vi "Modified Bartlett-Hanning Window.vi"   [LabVIEW 2020, in "NI_AALPro.lvlib"]
doc: "Applies a modified Bartlett-Hanning window to the input signal <B>X</B>. Wire data to the <B>X</B> input to determine the polymorphic instance to use or manually select the instance."
uses:
  <vilib>/Analysis/NI_AALPro.lvlib
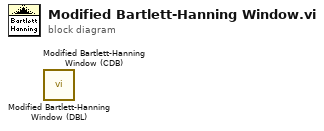
[diagram p0: block diagram]
diagram:
  n1 = call <vilib>:"Modified Bartlett-Hanning Window (DBL).vi"() -> ()  [unwired: 10 in, 2 out]
  n2 = call <vilib>:"Modified Bartlett-Hanning Window (CDB).vi"() -> ()  [unwired: 10 in, 2 out]
